vi "NIIE_Mouse Down_Tree.vi"(7 "Tree":refnum<vi>, 8 "Error":errorcluster, 11 "Coords":T1) -> (0 "Error Out":errorcluster)   [LabVIEW 2021]
uses:
  <vilib>/Utility/miscctls.llb/LVPoint32TypeDef.ctl
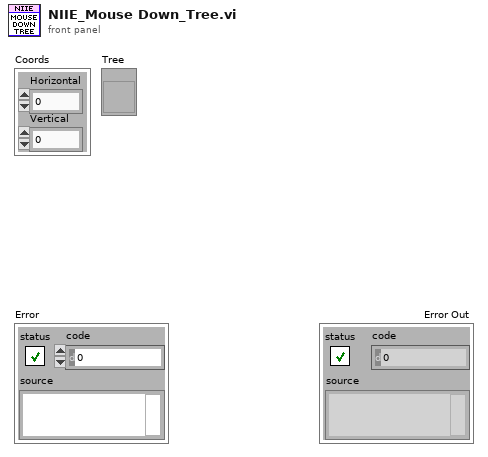
[diagram p1: front panel]
types:
  T1 = typedef "LVPoint32TypeDef.ctl" = cluster{"Horizontal":i32, "Vertical":i32}
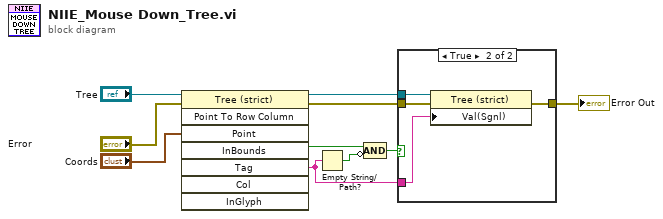
[diagram p0: block diagram]
diagram:
  n1 = invoke class="Tree (strict)" method="Point To Row Column"(reference="Tree", error in="Error", "Point"="Coords") -> (reference out=w7:refnum<vi>, error out=w6:errorcluster, "InBounds"=w3:bool, "Tag"=w1:string)  [unwired: 5 in, 4 out]
  n2 = Empty String/Path?(string/path=w1) -> (empty?=w4:bool)
  n3 = Compound Arithmetic op=AND(w3, invert w4) -> (w2:bool)
  n4 = case shown="True" w2 {
    tunnel: w7 -> [_ w15]
    tunnel: w6 -> [w11 w14]
    tunnel: [w11 w13] -> w5
    tunnel: w1 -> [_ w12]
    frame False {
    }
    frame True {
      n5 = property class="Tree (strict)"(reference=w15, error in=w14, "Val(Sgnl)"=w12) -> (error out=w13:errorcluster)  [unwired: 1 out]
    }
  }
  "Error Out" <- w5
